vi "Utility_Interpolate_V.vi"(9 "index":i32, 10 "length":i32, 11 "linear velocity":dbl) -> (3 "linear velocity":dbl)   [LabVIEW 2017]
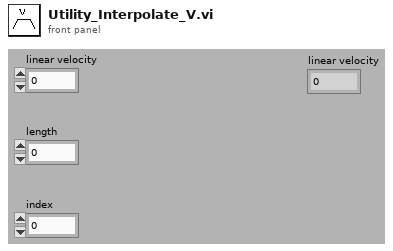
[diagram p1: front panel]
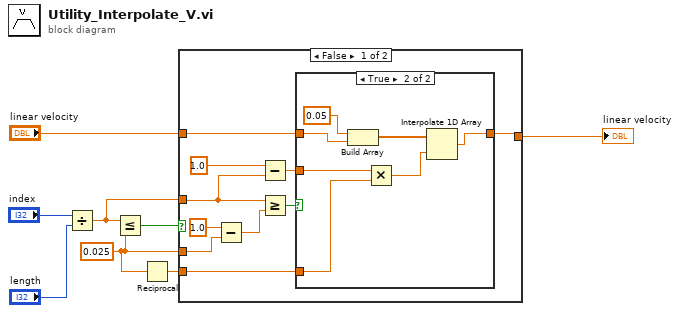
[diagram p0: block diagram]
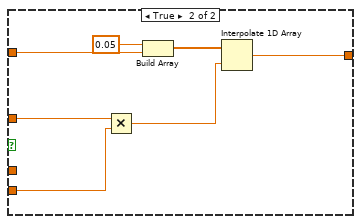
[diagram p3: hidden frame]
diagram:
  w1 = 0.025 ("y")
  n1 = Divide(x="index", y="length") -> (x/y=w6:dbl)
  n2 = Less Or Equal?(x=w6, y=w1) -> (x <= y?=w3:bool)
  n3 = Reciprocal(x=w1) -> (1/x=w2:dbl)
  n4 = case shown="False" w3 {
    tunnel: w6 -> [w14 w33]
    tunnel: "linear velocity" -> [w18 w32]
    tunnel: [w16 w28] -> w4
    tunnel: w2 -> [w9 w27]
    tunnel: w1 -> [w11 _]
    frame False {
      n5 = Subtract(x=1.0, y=w11) -> (x-y=w10:dbl)
      n6 = Subtract(x=1.0, y=w14) -> (x-y=w13:dbl)
      n7 = Greater Or Equal?(x=w14, y=w10) -> (x >= y?=w17:bool)
      n8 = case shown="True" w17 {
        tunnel: w18 -> [w19 w23]
        tunnel: [w19 w20] -> w16
        tunnel: w13 -> [_ w22]
        tunnel: w9 -> [_ w21]
        frame False {
        }
        frame True {
          n9 = Build Array(0.05 ("element"), w23) -> (w25:dbl[])
          n10 = Multiply(x=w22, y=w21) -> (x*y=w24:dbl)
          n11 = Interpolate 1D Array(1:w24, 2:w25) -> (0:w20:dbl)
        }
      }
    }
    frame True {
      n12 = Multiply(x=w33, y=w27) -> (x*y=w29:dbl)
      n13 = Build Array(0.05 ("element"), w32) -> (w30:dbl[])
      n14 = Interpolate 1D Array(1:w29, 2:w30) -> (0:w28:dbl)
    }
  }
  "linear velocity" <- w4
